vi "Add Items to Modified TypeDefs Tree.vi"(8 "error in":errorcluster, 10 "Dependent TypeDefs wParents":T1[](array[typedef]), 11 "TreeControl in":refnum<vi>) -> (0 "error out":errorcluster)   [LabVIEW 2013, in "DiscoverCommonTypeDefCallers.lvlib"]
uses:
  DiscoverCommonTypeDefCallers.lvlib
  Controls/DependendentTypeDefwParents.ctl
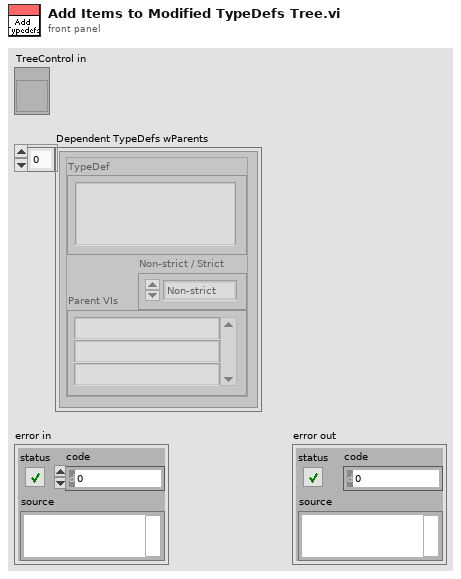
[diagram p1: front panel]
types:
  T1 = typedef "DiscoverCommonTypeDefCallers.lvlib/DependendentTypeDefwParents.ctl" = cluster{"TypeDef":string, "Non-strict / Strict":enum32{"Non-strict", "Strict"}, "Parent VIs":string[]}
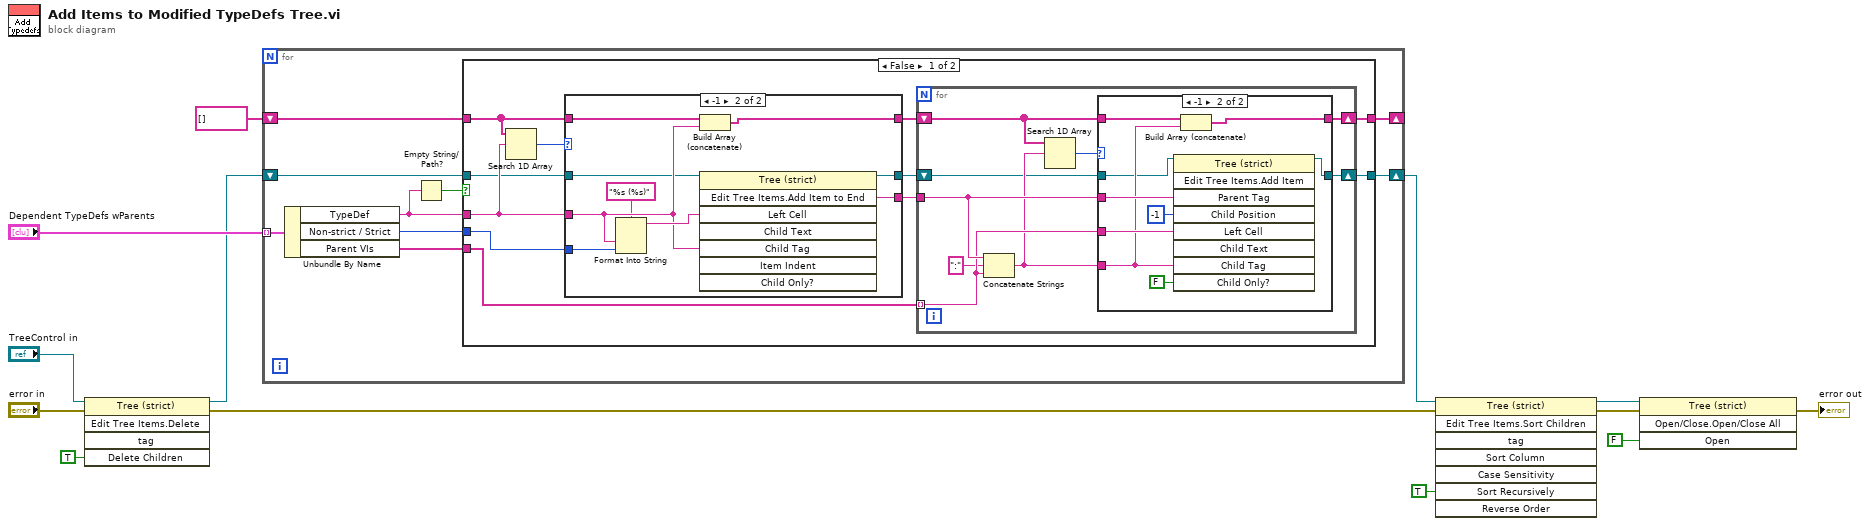
[diagram p0: block diagram]
diagram:
  n1 = invoke on="Invoke Node" class="Tree (strict)" method="Edit Tree Items.Delete"(reference="TreeControl in", error in="error in", "Delete Children"=TRUE ("Delete Children?")) -> (reference out=w4:refnum<vi>, error out=w3:errorcluster)  [unwired: 2 in, 3 out]
  n2 = for {
    tunnel: "Dependent TypeDefs wParents" -> [w22] mode=indexing
    shift-right: [w16] -> _
    shift-left: string[] [] ("Parent VIs") -> [w17]
    shift-right: [w14] -> w2
    shift-left: w4 -> [w15]
    n3 = Unbundle By Name(w22) -> ("TypeDef"=w19:string, "Non-strict / Strict"=w21:enum32{"Non-strict", "Strict"}, "Parent VIs"=w20:string[])
    n4 = Empty String/Path?(string/path=w19) -> (empty?=w18:bool)
    n5 = case shown="False" w18 {
      tunnel: w21 -> [w33 _]
      tunnel: w19 -> [w29 _]
      tunnel: w20 -> [w31 _]
      tunnel: w17 -> [w30 w67]
      tunnel: [w27 w67] -> w16
      tunnel: w15 -> [w25 w66]
      tunnel: [w23 w66] -> w14
      frame False {
        n6 = Search 1D Array(1D array=w30, element=w29) -> (index of element=w28:i32)  [unwired: 1 in]
        n7 = case shown="-1" w28 {
          tunnel: w33 -> [_ w45]
          tunnel: [w35 w44] -> w32
          tunnel: w30 -> [w36 w43]
          tunnel: w29 -> [w35 w40]
          tunnel: [w36 w42] -> w26
          tunnel: w25 -> [w34 w38]
          tunnel: [w34 w37] -> w24
          frame 0, Default {
          }
          frame -1 {
            n8 = Format Into String(format string="%s (%s)", w40, w45) -> (resulting string=w41:string)  [unwired: 2 in, 1 out]
            n9 = Build Array (concatenate)(w43, w40) -> (w42:string[])
            n10 = invoke on="Invoke Node" class="Tree (strict)" method="Edit Tree Items.Add Item to End"(reference=w38, "Left Cell"=w41, "Child Tag"=w40) -> (reference out=w37:refnum<vi>, "Edit Tree Items:Add Item to End"=w44:string)  [unwired: 5 in, 6 out]
          }
        }
        n11 = for {
          tunnel: w32 -> [w54]
          tunnel: w31 -> [w53] mode=indexing
          shift-right: [w50] -> w27
          shift-left: w26 -> [w51]
          shift-right: [w46] -> w23
          shift-left: w24 -> [w47]
          n12 = Concatenate Strings(w54, ":" ("string"), w53) -> (w49:string)
          n13 = Search 1D Array(1D array=w51, element=w49) -> (index of element=w48:i32)  [unwired: 1 in]
          n14 = case shown="-1" w48 {
            tunnel: w54 -> [_ w64]
            tunnel: w53 -> [_ w63]
            tunnel: w51 -> [w56 w62]
            tunnel: [w56 w61] -> w50
            tunnel: w49 -> [_ w60]
            tunnel: w47 -> [w55 w58]
            tunnel: [w55 w57] -> w46
            frame 0, Default {
            }
            frame -1 {
              n15 = invoke on="Invoke Node" class="Tree (strict)" method="Edit Tree Items.Add Item"(reference=w58, "Parent Tag"=w64, "Child Position"=-1, "Left Cell"=w63, "Child Tag"=w60, "Child Only?"=FALSE) -> (reference out=w57:refnum<vi>)  [unwired: 3 in, 8 out]
              n16 = Build Array (concatenate)(w62, w60) -> (w61:string[])
            }
          }
        }
      }
      frame True {
      }
    }
  }
  n17 = invoke on="Invoke Node" class="Tree (strict)" method="Edit Tree Items.Sort Children"(reference=w2, error in=w3, "Sort Recursively"=TRUE ("Sort Recursively?")) -> (reference out=w1:refnum<vi>, error out=w12:errorcluster)  [unwired: 5 in, 6 out]
  n18 = invoke on="Invoke Node" class="Tree (strict)" method="Open/Close.Open/Close All"(reference=w1, error in=w12, "Open"=FALSE ("Open?")) -> (error out=→"error out":errorcluster)  [unwired: 1 in, 3 out]
